vi "Add Button.vi"(8 "error in (no error)":errorcluster, 10 "Button":refnum<class "Button Interface.lvclass">, 11 "Basic Form in":refnum<class "Basic Form.lvclass">) -> (0 "error out":errorcluster, 3 "Basic Form out":refnum<class "Basic Form.lvclass">)   [LabVIEW 2020, in "Form.lvlib" / "Basic Form.lvclass"]
uses:
  Basic Form.lvclass
  Button Libraries/Button Interface Class/Button Interface.lvclass
  Basic Form.lvclass/Basic Form.ctl
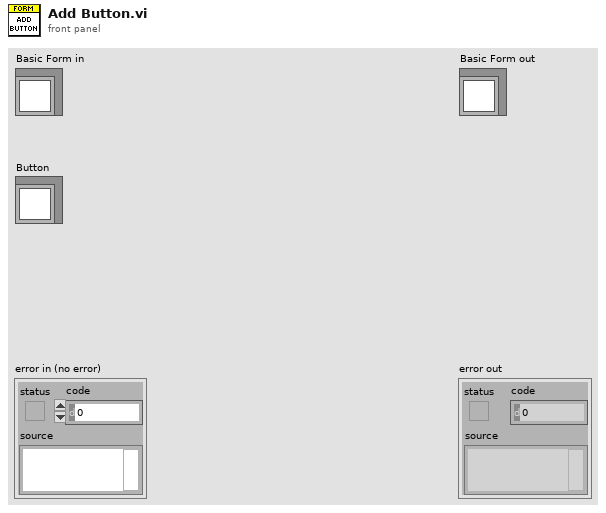
[diagram p1: front panel]
types:
  T1 = map{string, refnum<class "Button Interface.lvclass">}
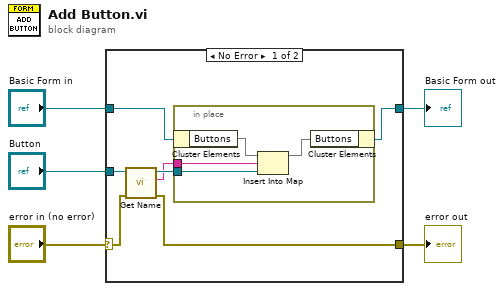
[diagram p0: block diagram]
diagram:
  n1 = case shown="No Error" "error in (no error)" {
    selector: "error in (no error)" -> [w7 w18]
    tunnel: [w6 w18] -> w4
    tunnel: [w8 w17] -> w2
    tunnel: "Basic Form in" -> [w11 w17]
    tunnel: "Button" -> [w12 _]
    frame No Error {
      n2 = call-dynamic "Get Name.vi"("error in (no error)"=w7, "Button Interface in"=w12) -> ("error out"=w6:errorcluster, "Name"=w9:string, "Button Interface out"=w10:refnum<class "Button Interface.lvclass">)  [unwired: 7 in]
      n3 = in-place {
        in-place-border: w10 -> [w14]
        in-place-border: w9 -> [w13]
        n4 = in-place-cluster #1(w11) -> ("Buttons"=w16:T1)
        n5 = Insert Into Map(map in=w16, key=w13, value=w14) -> (map out=w15:T1)  [unwired: 2 out]
        n6 = in-place-cluster #1("Buttons"=w15) -> (w8:refnum<class "Basic Form.lvclass">)
      }
    }
    frame Error {
    }
  }
  "error out" <- w4
  "Basic Form out" <- w2
